vi "find_pose.vi"(6 "Position valid":bool, 8 "Light positions":sgl[][](array[numeric]) format="%#.5f", 9 "XYZ index":i32=3, 10 "XYZ in":sgl[][](array[numeric]) format="%#.2f") -> (0 "Pose valid":bool, 2 "Pose":T1)   [LabVIEW 2013]
uses:
  <vilib>/Analysis/Matrix/Datatypes/RealMatrix.ctl
  <vilib>/Analysis/Matrix/NI_Matrix.lvlib
panel:
  in  "Max triad error":dbl=300.0
  # "Base index in XYZ for output or handle"
  # "Requires valid ASAP data, plus additional criteria related to pose."
  # "ASAP data valid"
  # "Parameters:"
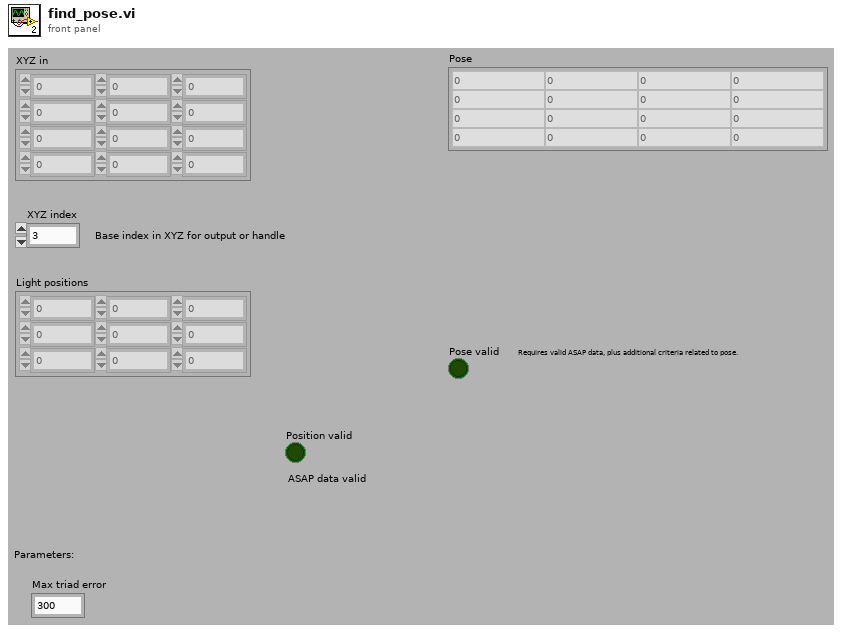
[diagram p1: front panel]
types:
  T1 = typedef "NI_Matrix.lvlib/RealMatrix.ctl" = dbl[][]
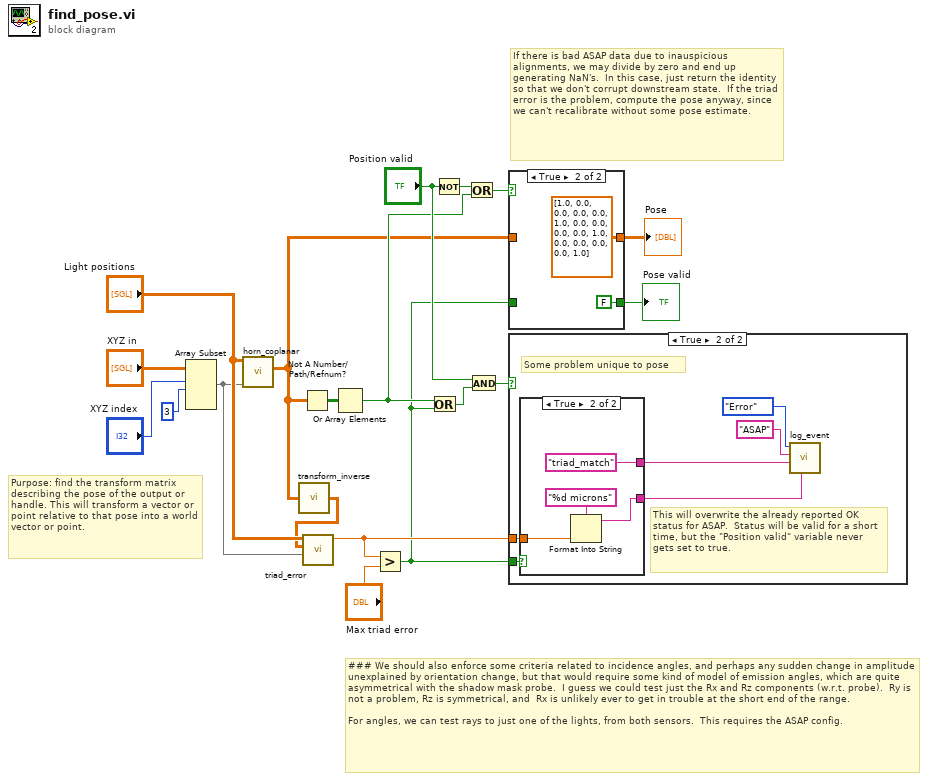
[diagram p0: block diagram]
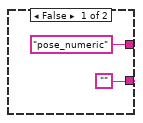
[diagram p3: hidden frame]
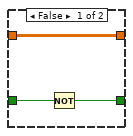
[diagram p4: hidden frame]
diagram:
  # "If there is bad ASAP data due to inauspicious alignments, we may divide by zero and end up generating NaN's.  In this case, just return the identity so that we don't corrupt downstream state.  If the triad error is the problem, compute the pose anyway, since we can't recalibrate without some pose estimate."
  # "### We should also enforce some criteria related to incidence angles, and perhaps any sudden change in amplitude unexplained by orientation change, but that would require some kind of model of emission angles, which are quite asymmetrical with the shadow mask probe.  I guess we could test just the Rx and Rz components (w.r.t. probe).  Ry is not a problem, Rz is symmetrical, and  Rx is unlikely ever to get in trouble at the short end of the range.\n\nFor angles, we can test rays to just one of the lights, from both sensors.  This requires the ASAP config."
  # "Purpose: find the transform matrix describing the pose of the output or handle. This will transform a vector or point relative to that pose into a world vector or point."
  n1 = Array Subset(array="XYZ in", index (row)="XYZ index", length (row)=3 ("length")) -> (w14:sgl[][])  [unwired: 2 in]
  n2 = call "horn_coplanar.vi"("Right points"=w14, "Left points"="Light positions") -> ("LR transform"=w2:T1)  [unwired: 9 out]
  n3 = call "transform_inverse.vi"("Transform"=w2) -> ("Inverse transform"=w1:T1)
  n4 = Not A Number/Path/Refnum?(number/path/refnum=w2) -> (NaN/Path/Refnum?=w17:bool[][])
  n5 = call "triad_error.vi"("Measured positions"=w14, "Measure transform"=w1, "Calibrated positions"="Light positions") -> ("RMS error"=w12:dbl)  [unwired: 7 in, 1 out]
  n6 = Or Array Elements(Boolean array=w17) -> (logical OR=w6:bool)
  n7 = Greater?(x=w12, y="Max triad error") -> (0:w4:bool)
  n8 = Or(x=w6, y=w4) -> (x .or. y?=w5:bool)
  n9 = Not(x="Position valid") -> (.not. x?=w9:bool)
  n10 = Or(x=w9, y=w6) -> (x .or. y?=w7:bool)
  n11 = And(x="Position valid", y=w5) -> (x .and. y?=w10:bool)
  n12 = case shown="True" w7 {
    tunnel: [w22 T1 [[1.0, 0.0, 0.0, 0.0], [0.0, 1.0, 0.0, 0.0], [0.0, 0.0, 1.0, 0.0], [0.0, 0.0, 0.0, 1.0]] ("LR transform")] -> w11
    tunnel: w2 -> [w22 _]
    tunnel: [w21 FALSE ("x .or. y?")] -> w3
    tunnel: w4 -> [w20 _]
    frame False {
      n13 = Not(x=w20) -> (.not. x?=w21:bool)
    }
    frame True {
    }
  }
  "Pose" <- w11
  "Pose valid" <- w3
  n14 = case shown="True" w10 {
    tunnel: w4 -> [_ w28]
    tunnel: w12 -> [_ w27]
    frame False {
    }
    frame True {
      # "This will overwrite the already reported OK status for ASAP.  Status will be valid for a short time, but the \"Position valid\" variable never gets set to true."
      # "Some problem unique to pose"
      n15 = case shown="True" w28 {
        tunnel: w27 -> [_ w34]
        tunnel: ["pose_numeric" ("Facility") "triad_match" ("Facility")] -> w26
        tunnel: ["" w33] -> w25
        frame False {
        }
        frame True {
          n16 = Format Into String(format string="%d microns", w34) -> (resulting string=w33:string)  [unwired: 2 in, 1 out]
        }
      }
      n17 = call "log_event.vi"("Message"=w25, "State"=w26, "Facility"="ASAP", "Severity"=enum16{"OK", "Debug", "Warn", "Error"}."Error") -> ()  [unwired: 7 in, 1 out]
    }
  }
